vi "Add Channel.vi"(8 "error in":errorcluster, 10 "channel":T1={"core"={"name"="Channel", "units"="V", "engine data type"=enum."DBL", "string data type"=enum."DBL", "string offset"=0}, "component settings"=[]} {"core"."string offset" format="%d bytes"}, 11 "transfer":T5={"core"={"name"="Transfer"}, "component settings"=[], "channels"=[]} {"channels"."core"."string offset" format="%d bytes"}) -> (0 "error out":errorcluster, 3 "transfer out":T5={"core"={"name"="Transfer"}, "component settings"=[], "channels"=[]} {"channels"."core"."string offset" format="%d bytes"})   [LabVIEW 2020, in "DSF Configuration API.lvlib"]
uses:
  DSF Configuration API.lvlib
  Includes/DSF Core.lvlibp/Typedefs/DSF Engine Transfer Configuration.ctl
  Includes/DSF Core.lvlibp/Typedefs/Core Transfer Configuration.ctl
  Includes/DSF Core.lvlibp/Typedefs/DSF Settings Info.ctl
  Includes/DSF Core.lvlibp/Typedefs/DSF Engine Channel Configuration.ctl
  Includes/DSF Core.lvlibp/Typedefs/Core Channel Configuration.ctl
  Includes/DSF Core.lvlibp/Typedefs/DSF Data Type.ctl
  Includes/DSF Core.lvlibp
  Includes/DSF Core.lvlibp/Classes/Configuration/Core/Channel/Channel Configuration.lvclass
  Includes/DSF Core.lvlibp/Classes/Configuration/Core/Transfer/Transfer Configuration.lvclass
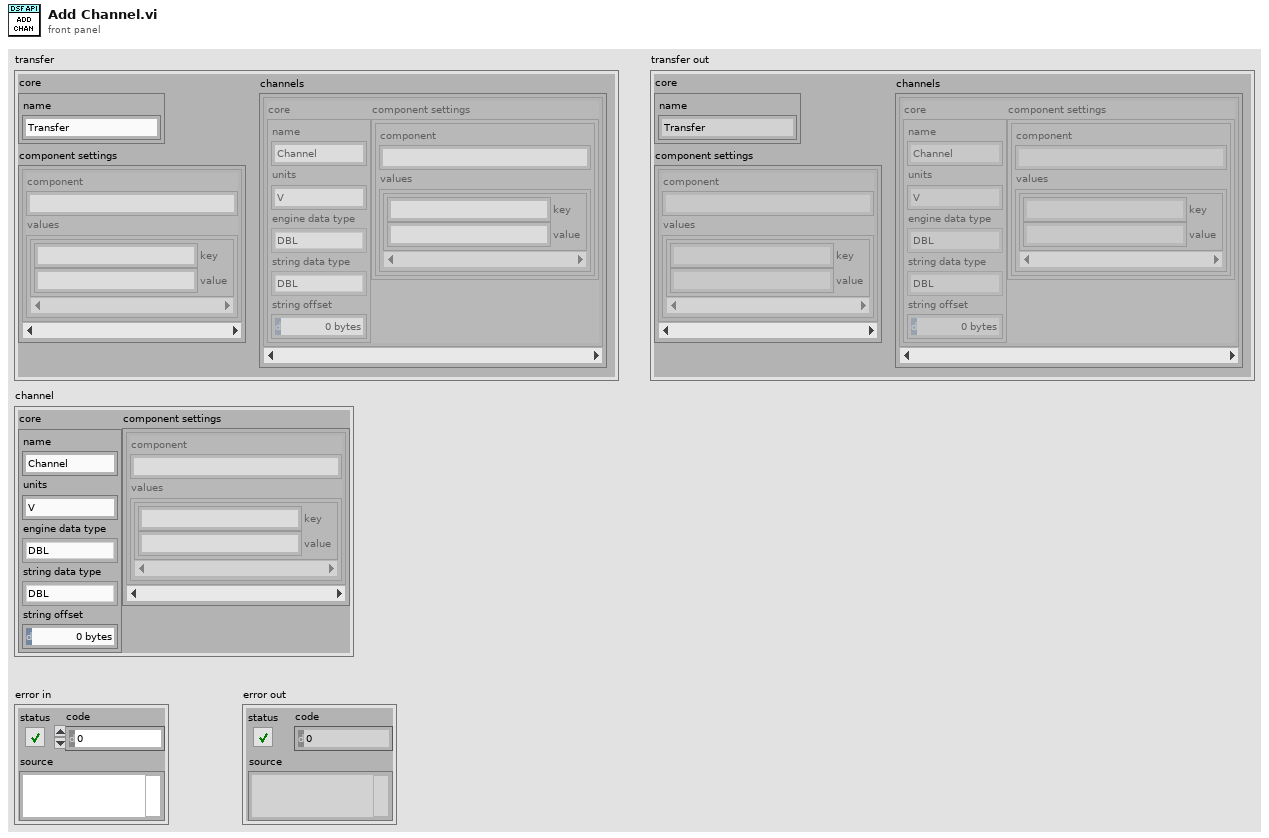
[diagram p1: front panel]
types:
  T1 = typedef "DSF Core.lvlibp/DSF Engine Channel Configuration.ctl" = cluster{"core":T2, "component settings":T4[]}
  T2 = typedef "DSF Core.lvlibp/Channel Configuration.lvclass/Core Channel Configuration.ctl" = cluster{"name":string, "units":string, "engine data type":T3, "string data type":T3, "string offset":u64}
  T3 = typedef "DSF Core.lvlibp/DSF Data Type.ctl" = enum8{"Bool", "SGL", "DBL", "I8", "I16", "I32", "I64", "U8", "U16", "U32", "U64"}
  T4 = typedef "DSF Core.lvlibp/DSF Settings Info.ctl" = cluster{"component":string, "values":cluster{"key":string, "value":string}[]}
  T5 = typedef "DSF Core.lvlibp/DSF Engine Transfer Configuration.ctl" = cluster{"core":T6, "component settings":T4[], "channels":T1[]}
  T6 = typedef "DSF Core.lvlibp/Transfer Configuration.lvclass/Core Transfer Configuration.ctl" = cluster{"name":string}
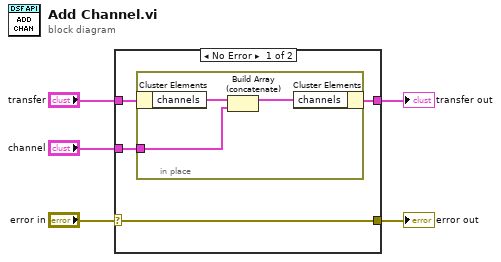
[diagram p0: block diagram]
diagram:
  n1 = case shown="No Error" "error in" {
    selector: "error in" -> [w7 w13]
    tunnel: "transfer" -> [w9 w14]
    tunnel: [w8 w14] -> w4
    tunnel: [w7 w13] -> w2
    tunnel: "channel" -> [w6 _]
    frame No Error {
      n2 = in-place {
        in-place-border: w6 -> [w10]
        n3 = in-place-cluster #1(w9) -> ("channels"=w12:T1[])
        n4 = Build Array (concatenate)(w12, w10) -> (w11:T1[])
        n5 = in-place-cluster #1("channels"=w11) -> (w8:T5)
      }
    }
    frame Error {
    }
  }
  "error out" <- w2
  "transfer out" <- w4
